vi "DataConversion.vi"(5 "Data In":dbl[][](array[numeric]) format="%0.2f", 6 "Init/Cont":bool) -> (0 "Blue Data":dbl[](array[numeric]), 1 "Pressure":dbl[](array[numeric]), 2 "Red Data":dbl[](array[numeric]), 3 "All Data":dbl[][](array[numeric]))   [LabVIEW 2013, in "main.lvlib"]
uses:
  main.lvlib
  Controls/Enum Variables.ctl
  <vilib>/Analysis/baseanly.llb/Mean (DBL).vi
  Globals/DataAcqRecordPathGlobal.vi
  <vilib>/Analysis/3filter.llb/Filter Passband Type.ctl
  <vilib>/Analysis/NI_AALBase.lvlib
  Controls/Enum Globals.ctl
  <vilib>/Analysis/3filter.llb/Zero Phase Filter (DBL).vi
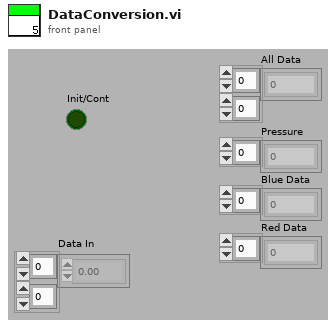
[diagram p1: front panel]
types:
  T1 = typedef "main.lvlib/Enum Variables.ctl" = enum16{"SetAcqFilter", "GetAcqFilter", "Set Filter", "Get Filter", "Set Height", "Get Height", "Set Recorded Height", "Get Recorded Height", "Set Blue Pressure", "Get Blue Pressure", "Set Red Pressure", "Get Red Pressure", "Init", "Reset Pressure", "Set Red Cursors", "Get Red Cursors", "Set Blue Cursors", "Get Blue Cursors", "Set Language", "Get Language", "Set Active Graphs", "Get ActiveGraphs", "Set Method", "Get Method", "Set Encryption", "Get Encryption", "Set ExcelVersion", "Get ExcelVersion", "Set DICOM Avail", "Get DICOM Avail", "Set DICOM Encode", "Get DICOM Encode", "Set JournalExport", "Get JournalExport", "Set Sequence", "Get Sequence", "Set DAQ Connected", "Get DAQ Connected", "Set Current Graph", "Get Current Graph", "Set General Settings", "Get Hyphenation", "Set Arm Calc Method", "Get Arm Calc Method", "Set Dicom Tags", "Get Dicom Tags", "Set BT Serial", "Get BT Serial", "Set BT Accepted Serials", "Get BT Accepted Serials", "Get BT License", "Set BT License"}
  T2 = typedef "main.lvlib/Enum Globals.ctl" = enum16{"Init", "Set DataPath", "Set Freq", "Get"}
  T3 = typedef "NI_AALBase.lvlib/Filter Passband Type.ctl" = enum32{"Lowpass", "Highpass", "Bandpass", "Bandstop"}
  T4 = cluster{"filter structure":enum32{"IIR 2nd Order", "IIR 4th Order"}, "Reverse Coefficients":dbl[], "Forward Coefficients":dbl[]}
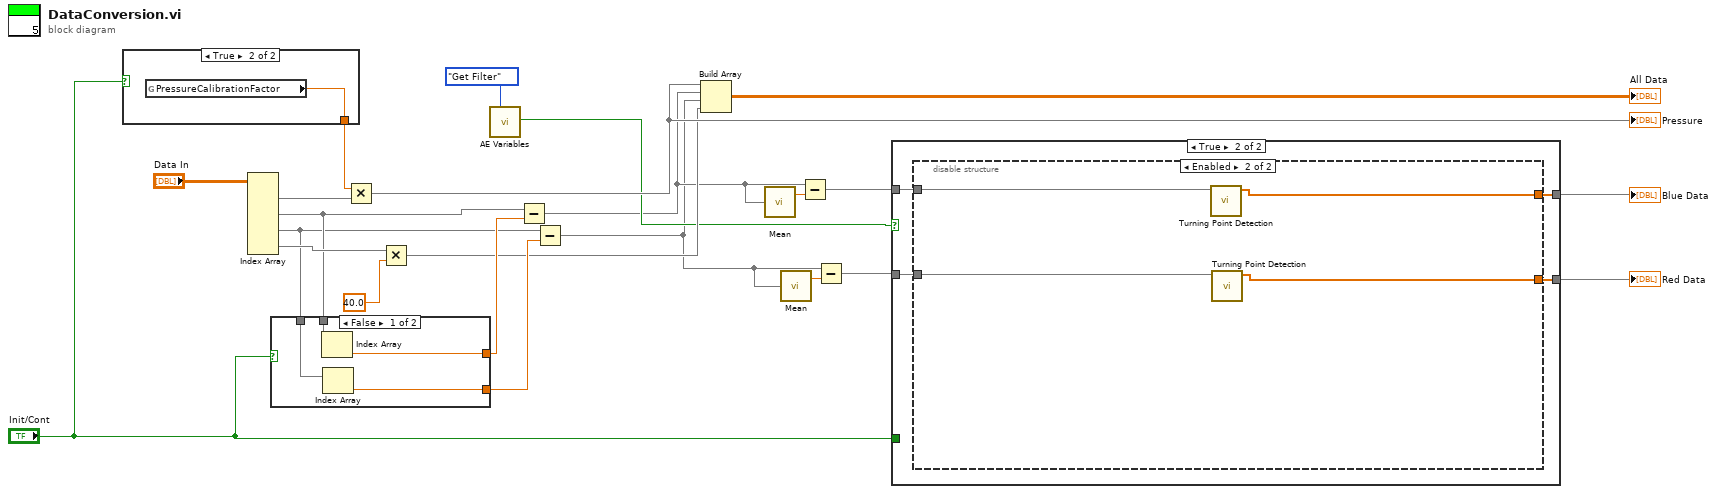
[diagram p0: block diagram]
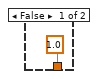
[diagram p2: hidden frame]
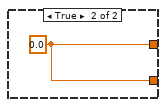
[diagram p3: hidden frame]
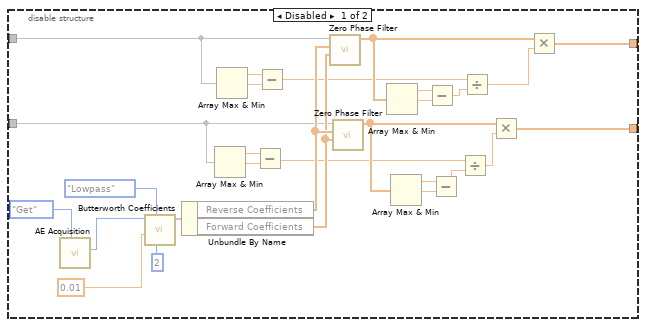
[diagram p5: hidden frame]
diagram:
  n1 = case shown="True" "Init/Cont" {
    tunnel: [1.0 ("PressureCalibrationFactor") w25] -> w16
    frame False {
    }
    frame True {
      n2 = global read "DataAcqRecordPathGlobal.vi" "PressureCalibrationFactor"() -> (w25:dbl)
    }
  }
  n3 = Index Array(array="Data In") -> (element #1=w23:dbl[], element #2=w15:dbl[], element #3=w14:dbl[], element #4=w21:dbl[])  [unwired: 8 in]
  n4 = case shown="False" "Init/Cont" {
    tunnel: w15 -> [w29 _]
    tunnel: [w28 w30] -> w18
    tunnel: w14 -> [w27 _]
    tunnel: [w26 w30] -> w17
    frame False {
      n5 = Index Array(array=w29) -> (element=w28:dbl)  [unwired: 1 in]
      n6 = Index Array(array=w27) -> (element=w26:dbl)  [unwired: 1 in]
    }
    frame True {
      w30 = 0.0 ("Waveform")
    }
  }
  n7 = Multiply(x=w16, y=w23) -> (x*y=w11:dbl[])
  "Pressure" <- w11
  n8 = Multiply(x=w21, y=40.0 ("Temperature Sensitivity")) -> (x*y=w10:dbl[])
  n9 = call "AE Variables.vi"("Action"=Enum_Variables."Get Filter") -> ("BooleanOut"=w9:bool)  [unwired: 11 in, 7 out]
  n10 = Subtract(x=w15, y=w18) -> (x-y=w4:dbl[])
  n11 = Subtract(x=w14, y=w17) -> (x-y=w2:dbl[])
  n12 = Build Array(w11, w4, w2, w10) -> (→"All Data":dbl[][])
  n13 = call-poly <vilib>:"Mean.vi"("X"=w4) -> ("mean"=w6:dbl)  [unwired: 1 out]
  n14 = call-poly <vilib>:"Mean.vi"("X"=w2) -> ("mean"=w3:dbl)  [unwired: 1 out]
  n15 = Subtract(x=w4, y=w6) -> (x-y=w5:dbl[])
  n16 = Subtract(x=w2, y=w3) -> (x-y=w1:dbl[])
  n17 = case shown="True" w9 {
    tunnel: w1 -> [w31 w33]
    tunnel: w5 -> [w32 w34]
    tunnel: [w32 w35] -> w8
    tunnel: [w31 w36] -> w7
    tunnel: "Init/Cont" -> [_ _]
    frame False {
    }
    frame True {
      n18 = disable-structure shown="Enabled" {
        disable-tunnel: [w56 w65] -> w36
        disable-tunnel: [w55 w67] -> w35
        disable-tunnel: w34 -> [w54 w68]
        disable-tunnel: w33 -> [w49 w66]
        frame Disabled {
          n19 = call "AE Acquisition.vi"("Action"=Enum_Globals."Get") -> ("Freq Out"=w57:i32)  [unwired: 7 in, 3 out]
          n20 = call <vilib>:"Butterworth Coefficients.vi"("order"=2, "filter type"=Filter_Passband_Type."Lowpass", "low cutoff freq: fl"=0.01, "sampling freq: fs"=w57) -> ("IIR Filter Cluster"=w64:T4)  [unwired: 6 in, 1 out]
          n21 = Unbundle By Name(w64) -> ("Reverse Coefficients"=w60:dbl[], "Forward Coefficients"=w59:dbl[])
          n22 = Array Max & Min(array=w49) -> (max value=w51:dbl, min value=w50:dbl)  [unwired: 2 out]
          n23 = Array Max & Min(array=w54) -> (max value=w53:dbl, min value=w52:dbl)  [unwired: 2 out]
          n24 = Subtract(x=w51, y=w50) -> (x-y=w38:dbl)
          n25 = Subtract(x=w53, y=w52) -> (x-y=w42:dbl)
          n26 = call-poly <vilib>:"Zero Phase Filter.vi"("Forward Coefficients"=w59, "Reverse Coefficients"=w60, "X"=w54) -> ("Filtered X"=w43:dbl[])  [unwired: 7 in, 1 out]
          n27 = call-poly <vilib>:"Zero Phase Filter.vi"("Forward Coefficients"=w59, "Reverse Coefficients"=w60, "X"=w49) -> ("Filtered X"=w46:dbl[])  [unwired: 7 in, 1 out]
          n28 = Array Max & Min(array=w43) -> (max value=w45:dbl, min value=w44:dbl)  [unwired: 2 out]
          n29 = Array Max & Min(array=w46) -> (max value=w48:dbl, min value=w47:dbl)  [unwired: 2 out]
          n30 = Subtract(x=w45, y=w44) -> (x-y=w41:dbl)
          n31 = Subtract(x=w48, y=w47) -> (x-y=w39:dbl)
          n32 = Divide(x=w38, y=w39) -> (x/y=w37:dbl)
          n33 = Divide(x=w42, y=w41) -> (x/y=w40:dbl)
          n34 = Multiply(x=w46, y=w37) -> (x*y=w56:dbl[])
          n35 = Multiply(x=w43, y=w40) -> (x*y=w55:dbl[])
        }
        frame Enabled {
          n36 = call "Turning Point Detection.vi"("Input"=w68) -> ("Best BSpline Fit"=w67:dbl[])  [unwired: 9 in, 1 out]
          n37 = call "Turning Point Detection.vi"("Input"=w66) -> ("Best BSpline Fit"=w65:dbl[])  [unwired: 9 in, 1 out]
        }
      }
    }
  }
  "Blue Data" <- w8
  "Red Data" <- w7
